vi "ErrorSubUI.vi"() -> ()   [LabVIEW 2016]
uses:
  Package ResourceControl/ViHandler/ViHandler.ViInfo.ctl
  Package Libraries/Message Queue/private/MessageQueue.MessageTypeDef.ctl
  Package ErrorHandling/ErrorHandling.lvclass/ErrorHandling.ctl
  Package Libraries/StringFunctions/StringFunctions_ReplaceAllBlindSigns.vi
  Package ErrorHandling/ErrorHandling.checkForErrorAndHandle.vi
  <vilib>/dlg_ctls.llb/Space Constant.vi
  <vilib>/Utility/error.llb/Clear Errors.vi
  <vilib>/Utility/error.llb/Trim Whitespace.vi
  <vilib>/Utility/error.llb/Search and Replace Pattern.vi
  <vilib>/Utility/error.llb/Error Cluster From Error Code.vi
  Package Libraries/TimingFunctions/TimingFunctions_getUtcTimestamp.vi
  Package ErrorHandling/ErrorHandling.addLastErrorToFile.vi
  Package ErrorHandling/ErrorHandling.lvclass
  <vilib>/ErrorRing/Error Ring.xnode
  Package ResourceControl/ViHandler/ViHandler.lvclass
panel:
  in  "PauseBtn":bool
  in  "ClearErrorHistoryBtn":bool
  in  "ErrorList":i32(listbox)
  out "EndOfBuffer[ms]":u32
  out "ViInfoTemp":T1
  # "(Error Logging will still be contiuned in the background)"
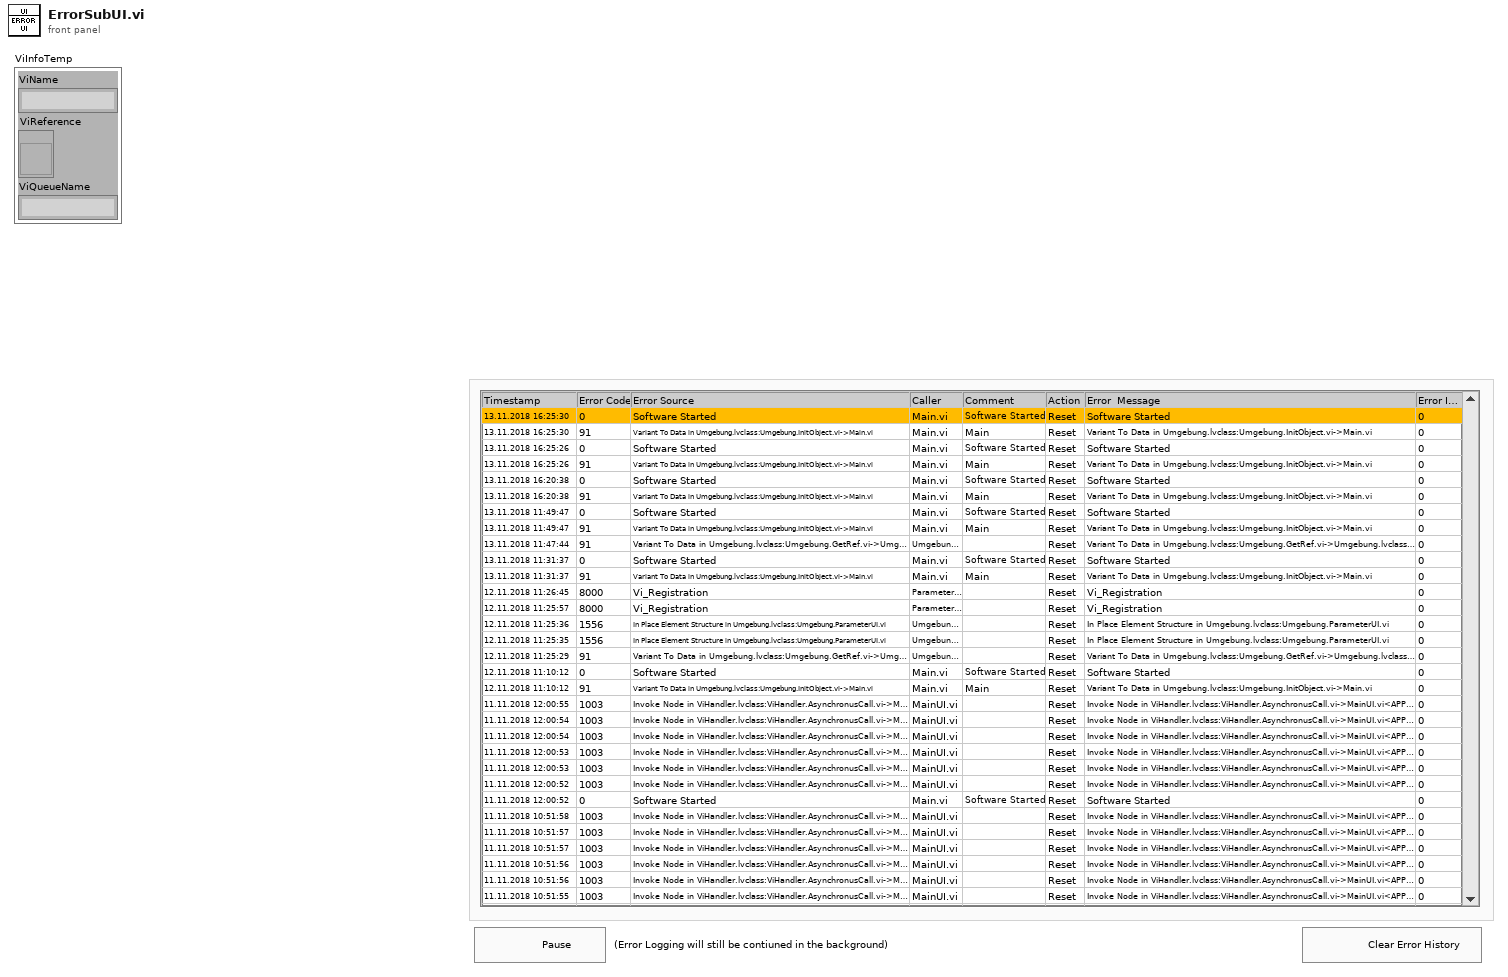
[diagram p1: front panel]
types:
  T1 = typedef "ViHandler.lvclass/ViHandler.ViInfo.ctl" = cluster{"ViName":string, "ViReference":refnum<vi>, "ViQueueName":string}
  T2 = typedef "MessageQueue.MessageTypeDef.ctl" = cluster{"Message":string, "Data":variant}
  T3 = typedef "ErrorHandling.lvclass/ErrorHandling.OccurredErrorDataStruct.ctl" = cluster{"Error":errorcluster, "Caller":string, "Comment":string, "Timestamp":timestamp, "Stopped":bool, "ErrorCusterString":string, "ErrorIndex":u64}
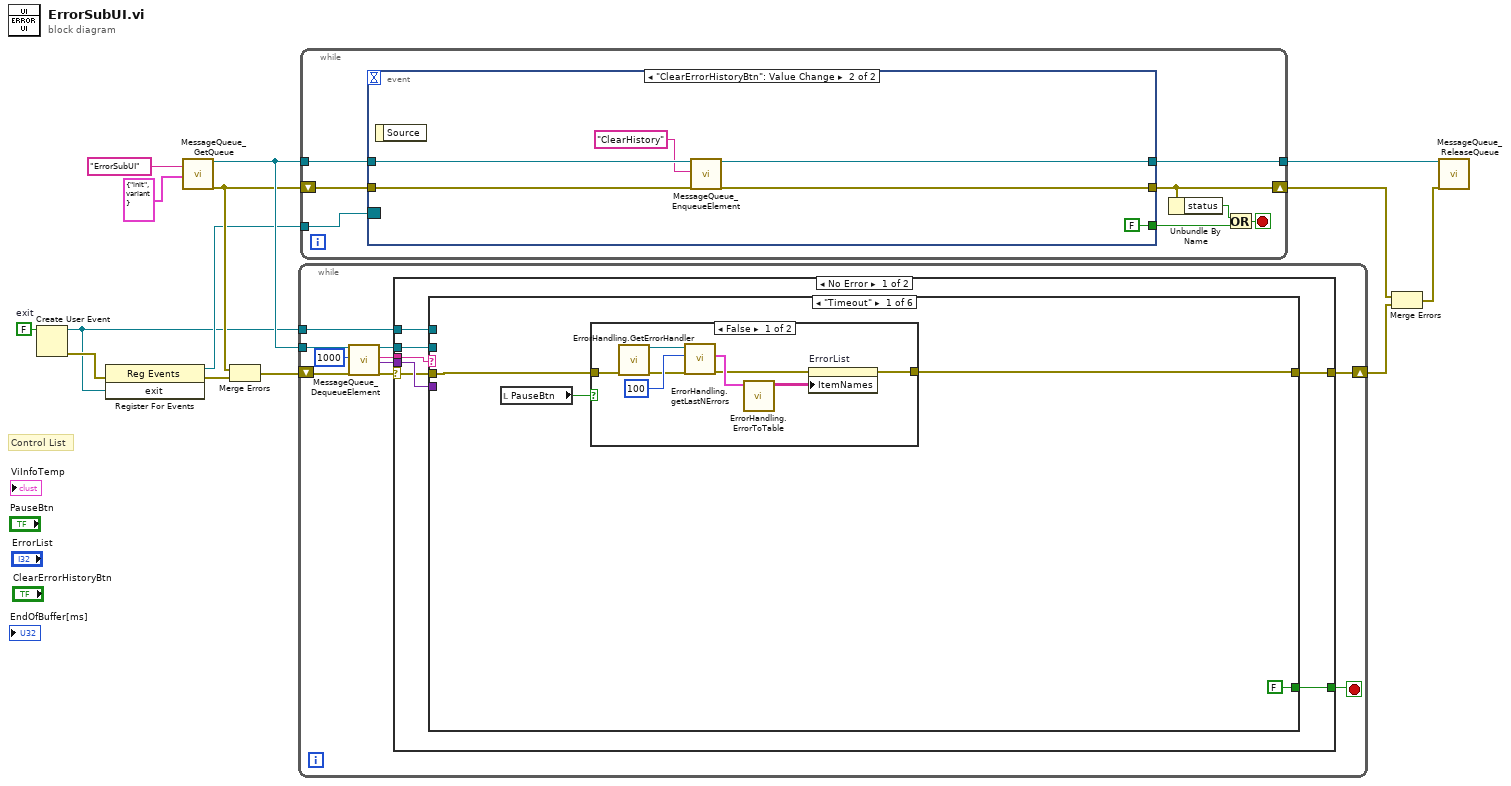
[diagram p0: block diagram]
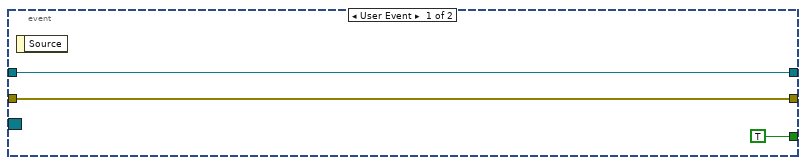
[diagram p2: hidden frame]
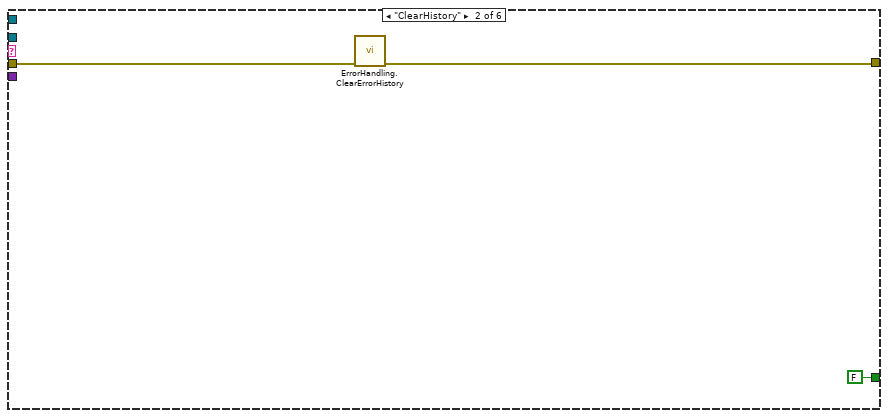
[diagram p4: hidden frame]
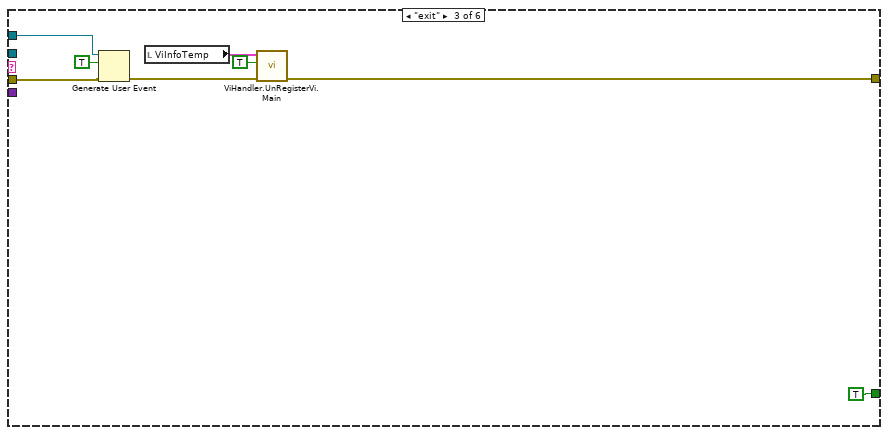
[diagram p5: hidden frame]
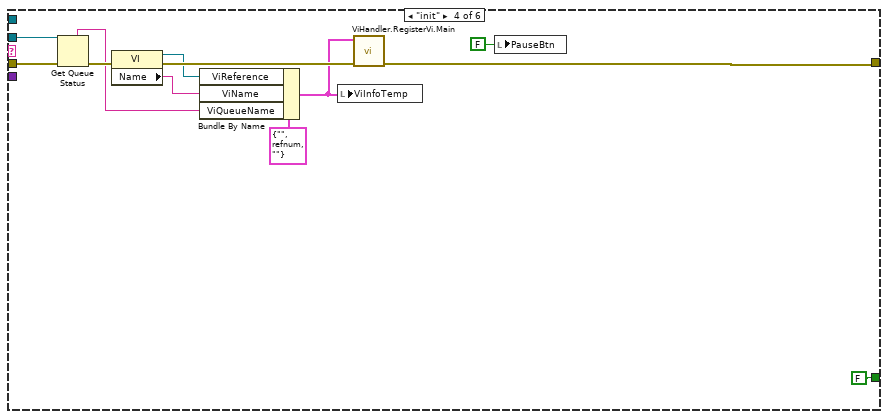
[diagram p6: hidden frame]
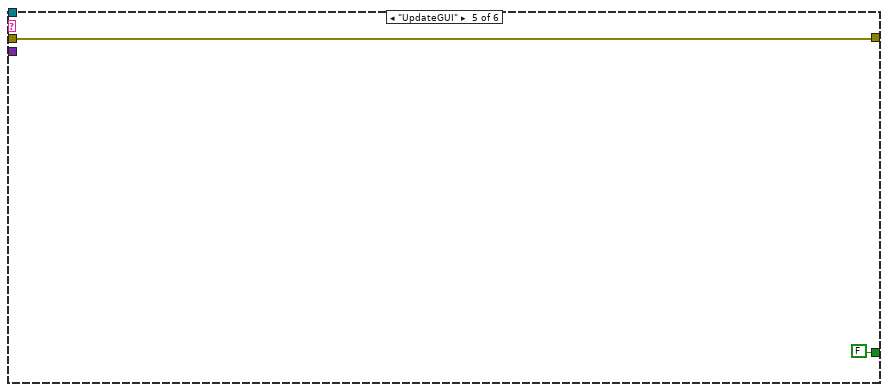
[diagram p7: hidden frame]
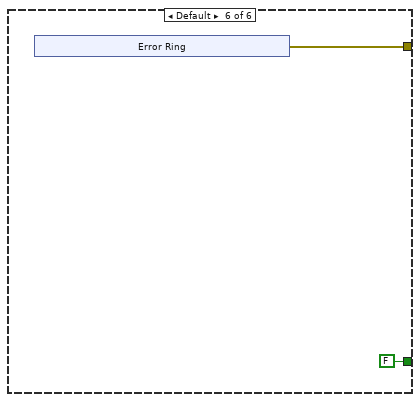
[diagram p8: hidden frame]
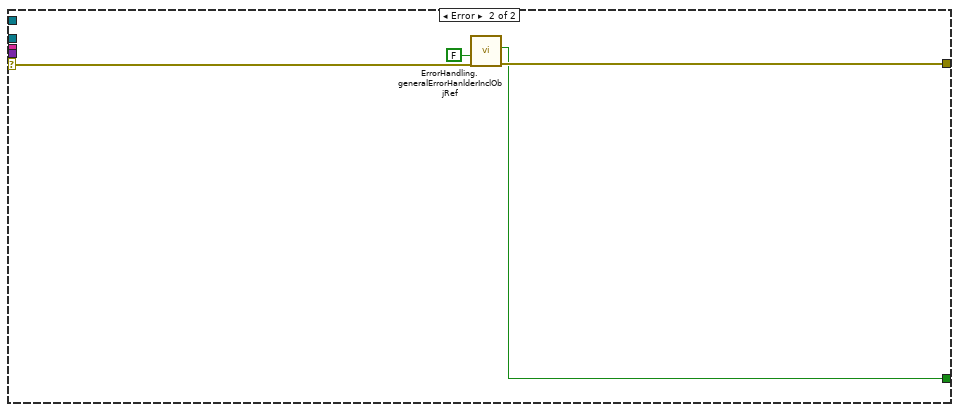
[diagram p9: hidden frame]
diagram:
  w7 = FALSE  # exit
  # "Control List"
  n1 = Create User Event(user event datatype=w7) -> (user event=w5:refnum<user-event>, error out=w6:errorcluster)  [unwired: 1 in]
  n2 = register-events(error in=w6, w5) -> (reference out=w9:refnum<event-registration>, error out=w11:errorcluster)  [unwired: 1 in]
  n3 = call "MessageQueue_GetQueue.vi"("Name"="ErrorSubUI", "OptionalInitValue"=T2 {"Message"="init", "Data"=variant}) -> ("QueueOut"=w13:refnum<queue>, "ErrorOut"=w10:errorcluster)  [unwired: 15 in, 1 out]
  n4 = Merge Errors(w10, w11) -> (w8:errorcluster)
  n5 = while {
    tunnel: w13 -> [w24]
    tunnel: w5 -> [w17]
    shift-right: [w16] -> w3
    shift-left: w8 -> [w18]
    stop <- w19 stop-if-true
    n6 = call "MessageQueue_DequeueElement.vi"("QueueIn"=w24, "Timeout"=1000, "ErrorIn"=w18) -> ("QueueOut"=w22:refnum<queue>, "Message"=w21:string, "Data"=w20:variant, "ErrorOut"=w23:errorcluster)  [unwired: 12 in, 1 out]
    n7 = case shown="No Error" w23 {
      selector: w23 -> [w27 w80]
      tunnel: w22 -> [w31 _]
      tunnel: w21 -> [w30 _]
      tunnel: w20 -> [w29 _]
      tunnel: [w28 w78] -> w19
      tunnel: w17 -> [w26 _]
      tunnel: [w25 w79] -> w16
      frame No Error {
        n8 = case shown="\"Timeout\"" w30 {
          tunnel: w31 -> [_ _ _ w61 _ _]
          tunnel: w29 -> [_ _ _ _ _ _]
          tunnel: [FALSE FALSE TRUE FALSE FALSE FALSE] -> w28
          tunnel: w27 -> [w34 w46 w53 w58 w68 _]
          tunnel: w26 -> [_ _ w52 _ _ _]
          tunnel: [w33 w45 w49 w57 w68 w71] -> w25
          frame "Timeout" {
            n9 = local read "PauseBtn"() -> (w32:bool)
            n10 = case shown="False" w32 {
              tunnel: w34 -> [w40 w44]
              tunnel: [w36 w44] -> w33
              frame False {
                n11 = call "ErrorHandling.GetErrorHandler.vi"("ErrorIn"=w40) -> ("ErrorOut"=w41:errorcluster, "ErrorRef"=w43:refnum<data-value>)  [unwired: 8 in, 1 out]
                n12 = call "ErrorHandling.getLastNErrors.vi"("error in (no error)"=w41, "N"=u32 100, "ErrorHandling in"=w43) -> ("error out"=w37:errorcluster, "Errors"=w39:T3[])  [unwired: 6 in, 1 out]
                n13 = call "ErrorHandling.ErrorToTable.vi"("Errors"=w39) -> ("Item Names"=w38:string[][])  [unwired: 10 in]
                n14 = property on="ErrorList" class="MCListbox (strict)"(error in=w37, "ItemNames"=w38) -> (error out=w36:errorcluster)  [unwired: 1 in, 1 out]
              }
              frame True {
              }
            }
          }
          frame "ClearHistory" {
            n15 = call "ErrorHandling.ClearErrorHistory.vi"("error IO"=w46) -> ("error IO"=w45:errorcluster)  [unwired: 10 in]
          }
          frame "exit" {
            n16 = Generate User Event(user event=w52, event data cluster=TRUE ("event data"), error in=w53) -> (error out=w50:errorcluster)  [unwired: 1 in, 1 out]
            n17 = local read "ViInfoTemp"() -> (w51:T1)
            n18 = call "ViHandler.UnRegisterVi.Main.vi"("ErrorIn"=w50, "FinalExit?"=TRUE, "ViInfo"=w51) -> ("ErrorOut"=w49:errorcluster)  [unwired: 7 in, 1 out]
          }
          frame "init" {
            n19 = Get Queue Status(queue=w61, error in (no error)=w58) -> (queue name=w59:string, error out=w65:errorcluster)  [unwired: 1 in, 6 out]
            n20 = property class="VI"(error in=w65) -> (reference out=w63:refnum<vi>, error out=w64:errorcluster, "Name"=w62:string)  [unwired: 1 in]
            n21 = Bundle By Name(cluster=T1 {"ViName"="", "ViReference"=refnum, "ViQueueName"=""} ("ViInfo"), "ViReference"=w63, "ViName"=w62, "ViQueueName"=w59) -> (w60:T1)
            n22 = local write "ViInfoTemp"(w60) -> ()
            n23 = call "ViHandler.RegisterVi.Main.vi"("ErrorIn"=w64, "ViInfo"=w60) -> ("ErrorOut"=w57:errorcluster)  [unwired: 9 in]
            n24 = local write "PauseBtn"(FALSE ("PauseBtn")) -> ()
          }
          frame "UpdateGUI" {
          }
          frame Default {
            n25 = xnode "Error Ring"() -> ("error out"=w71:errorcluster)
          }
        }
      }
      frame Error {
        n26 = call "ErrorHandling.generalErrorHanlderInclObjRef.vi"("error in"=w80, "StopOnError"=FALSE) -> ("error out"=w79:errorcluster, "Stop"=w78:bool)  [unwired: 7 in, 1 out]
      }
    }
  }
  n27 = while {
    tunnel: w13 -> [w88]
    tunnel: [w87] -> w14
    shift-right: [w84] -> w2
    shift-left: w10 -> [w86]
    tunnel: w9 -> [w81]
    stop <- w83 stop-if-true
    n28 = event shown="[1] \"ClearErrorHistoryBtn\": Value Change" {
      selector: w81 -> [_ _]
      dyn-events: _ -> [_ _]
      timeout: _ -> [_ _]
      tunnel: w88 -> [w90 w97]
      tunnel: [w90 w94] -> w87
      tunnel: [w89 w95] -> w84
      tunnel: w86 -> [w89 w96]
      tunnel: [TRUE FALSE] -> w85
      event User Event {
        n29 = event-data() -> ()  [unwired: 1 in, 1 out]
      }
      event "ClearErrorHistoryBtn": Value Change {
        n30 = event-data() -> ()  [unwired: 1 in, 1 out]
        n31 = call "MessageQueue_EnqueueElement.vi"("QueueIn"=w97, "Message"="ClearHistory", "ErrorIn"=w96) -> ("QueueOut"=w94:refnum<queue>, "ErrorOut"=w95:errorcluster)  [unwired: 15 in]
      }
    }
    n32 = Unbundle By Name(w84) -> ("status"=w82:bool)
    n33 = Or(x=w82, y=w85) -> (x .or. y?=w83:bool)
  }
  n34 = Merge Errors(w2, w3) -> (w1:errorcluster)
  n35 = call "MessageQueue_ReleaseQueue.vi"("QueueIn"=w14, "ErrorIn"=w1) -> ()  [unwired: 15 in, 3 out]
